vi "vision-board.vi"(8 "error in":errorcluster) -> (0 "error out":errorcluster, 2 "recycle?":bool, 3 "vision board":T2)   [LabVIEW 2019]
uses:
  vision_board_ctl.ctl
panel:
  out "Image Out 3":T1(plugin-control)
  out "Array":string[][](array[string])
  out "Image Out 2":T1(plugin-control)
  out "recycle index":i32
  out "Image Out":T1(plugin-control)
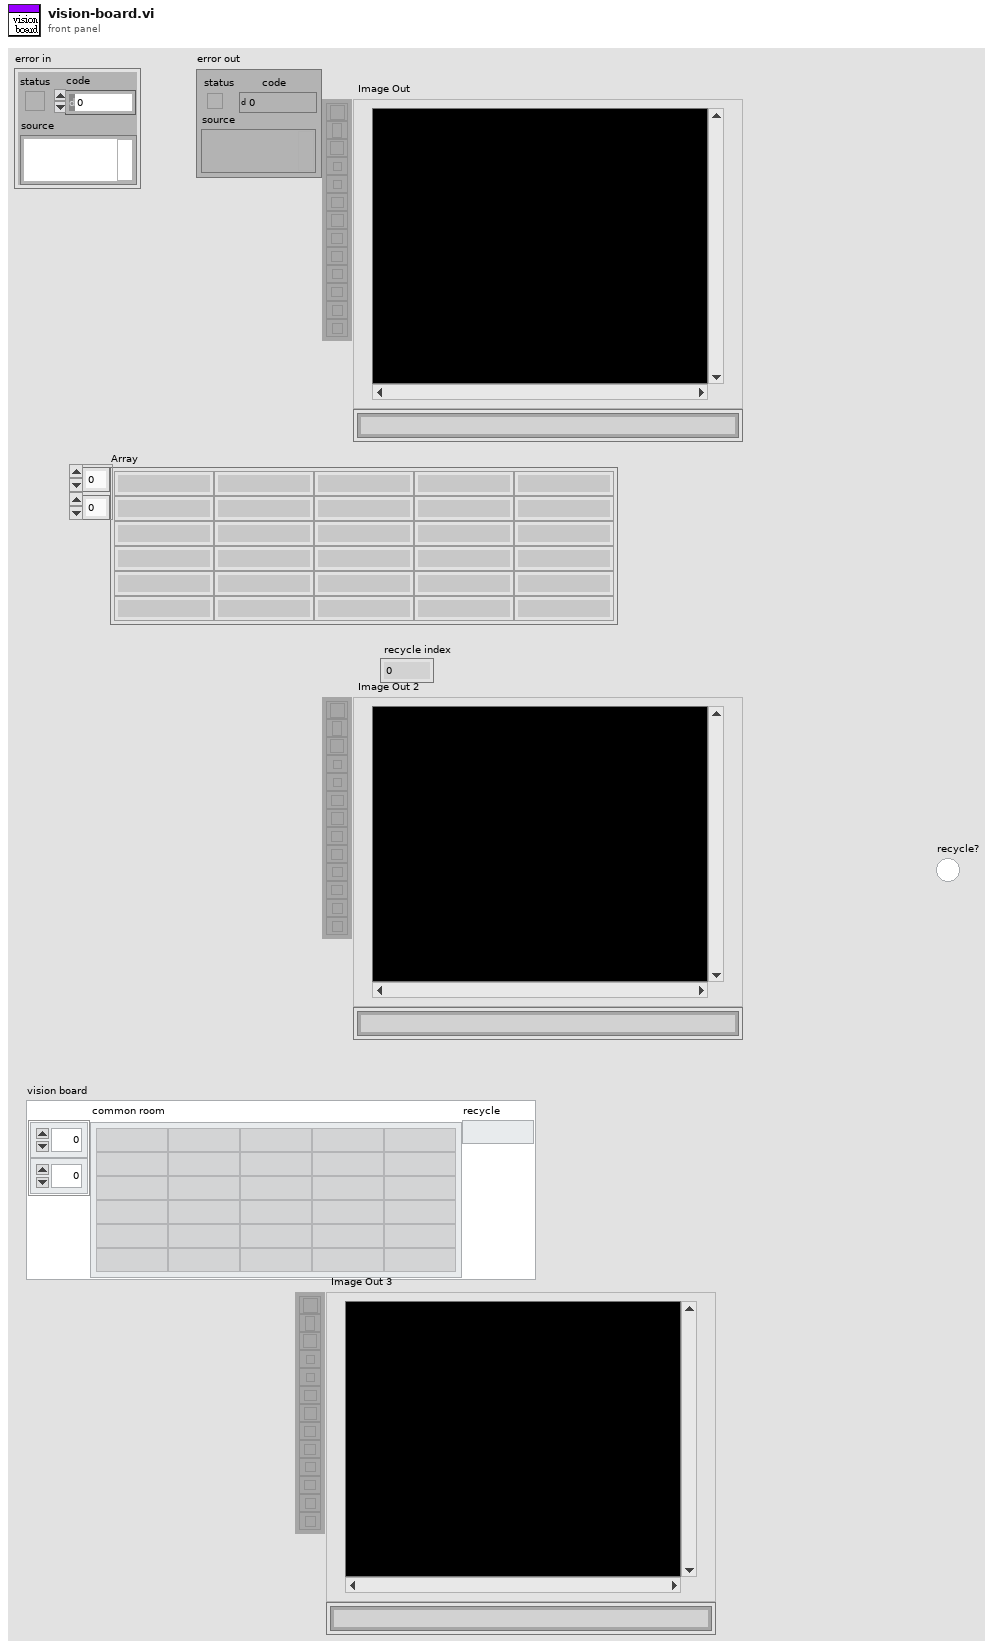
[diagram p1: front panel]
types:
  T1 = typedef "IMAQ Image.ctl" = refnum<image>
  T2 = typedef "vision_board_ctl.ctl" = cluster{"common room":string[][], "recycle":string}
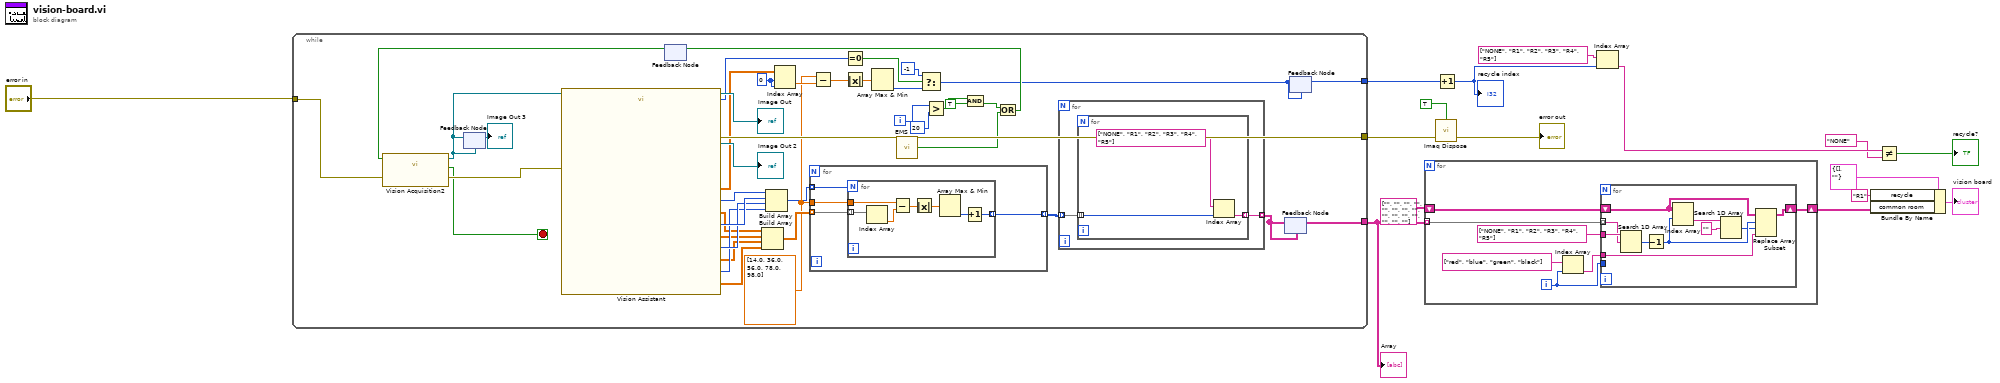
[diagram p0: block diagram]
diagram:
  n1 = while {
    tunnel: [w22] -> w16
    tunnel: "error in" -> [w32]
    tunnel: [w52] -> w4
    tunnel: [w24] -> w15
    i -> [w29]
    stop <- w20 stop-if-true
    w39 = sgl[] [14.0, 36.0, 56.0, 78.0, 98.0] ("Array")
    w55 = 0 ("length")
    n2 = feedback #1() -> (w25:bool)  [unwired: 1 in]
    n3 = call "Vision Acquisition2"("Stop (F)"=w25, "error in"=w32) -> ("Image Out"=w18:T1, "Stopped"=w20:bool, "error out"=w31:errorcluster)  [unwired: 23 in]
    n4 = feedback-in #2(w18) -> ()
    n5 = feedback #2(w18) -> (→"Image Out 3":T1)
    n6 = call "Vision Assistant"("Image In"=w18, "error in"=w31) -> ("Number of Particles (black)"=w45:i32, "Number of Particles (green)"=w46:i32, "Number of Particles (Blue)"=w47:i32, "Number of Particles (red)"=w48:i32, "Image Buffer (Image Buffer 5)"=→"Image Out 2":T1, "Image Out"=→"Image Out":T1, "Number of Particles (Yellow)"=w34:i32, "Particle Measurements (Pixels) (Yellow)"=w38:dbl[][], "Particle Measurements (Pixels) (red)"=w44:dbl[][], "Particle Measurements (Pixels) (Blue)"=w41:dbl[][], "Particle Measurements (Pixels) (green)"=w42:dbl[][], "Particle Measurements (Pixels) (black)"=w43:dbl[][], "error out"=w52:errorcluster)  [unwired: 13 in]
    n7 = Build Array(w44, w41, w42, w43) -> (w40:dbl[][][])
    n8 = Build Array(w48, w47, w46, w45) -> (w33:i32[])
    n9 = Index Array(array=w38, index (row)=w55, index (col)=w55) -> (element=w54:dbl)
    n10 = for {
      tunnel: w33 -> [w66] mode=indexing
      tunnel: w40 -> [w65] mode=indexing
      tunnel: w39 -> [w64]
      tunnel: [w63] -> w35 mode=indexing
      n11 = for {
        N: w66 -> [_]
        tunnel: w65 -> [w73] mode=indexing
        tunnel: w64 -> [w72]
        tunnel: [w67] -> w63 mode=indexing
        n12 = Index Array(array=w73) -> (element=w71:dbl)  [unwired: 1 in]
        n13 = Subtract(x=w72, y=w71) -> (x-y=w69:dbl[])
        n14 = Absolute Value(x=w69) -> (abs(x)=w70:dbl[])
        n15 = Array Max & Min(array=w70) -> (min index (indices)=w68:i32)  [unwired: 3 out]
        n16 = Increment(x=w68) -> (x+1=w67:i32)
      }
    }
    n17 = Subtract(x=w39, y=w54) -> (x-y=w57:dbl[])
    n18 = Equal To 0?(x=w34) -> (x = 0?=w37:bool)
    n19 = Absolute Value(x=w57) -> (abs(x)=w56:dbl[])
    n20 = Array Max & Min(array=w56) -> (min index (indices)=w53:i32)  [unwired: 3 out]
    n21 = call "EMS.vi"() -> ("A/DIO4 (Pin 19)"=w51:bool)
    n22 = Select(t=-1, s=w37, f=w53) -> (s? t:f=w21:i32)
    n23 = Greater?(x=w29, y=20) -> (0:w27:bool)
    n24 = And(x=w27, y=TRUE) -> (x .and. y?=w30:bool)
    n25 = Or(x=w30, y=w51) -> (x .or. y?=w26:bool)
    n26 = feedback-in #1(w26) -> ()
    n27 = for {
      tunnel: w35 -> [w58] mode=indexing
      tunnel: [w59] -> w23 mode=indexing
      n28 = for {
        tunnel: w58 -> [w61] mode=indexing
        tunnel: [w60] -> w59 mode=indexing
        n29 = Index Array(array=string[] ["NONE", "R1", "R2", "R3", "R4", "R5"], index=w61) -> (element=w60:string)
      }
    }
    n30 = feedback-in #3(w23) -> ()
    n31 = feedback #3(w23) -> (w24:string[][])
    n32 = feedback-in #4(w21) -> ()
    n33 = feedback #4(w21) -> (w22:i32)
  }
  "Array" <- w15
  n34 = for {
    tunnel: w15 -> [w80] mode=indexing
    shift-right: [w74] -> w13
    shift-left: string[][] [["", "", ""], ["", "", ""], ["", "", ""], ["", "", ""], ["", "", ""]] -> [w75]
    i -> [w76]
    n35 = Index Array(array=string[] ["red", "blue", "green", "black"], index=w76) -> (element=w77:string)
    n36 = for {
      tunnel: w80 -> [w89] mode=indexing
      tunnel: string[] ["NONE", "R1", "R2", "R3", "R4", "R5"] -> [w90]
      tunnel: w77 -> [w82]
      tunnel: w76 -> [_]
      shift-right: [w81] -> w74
      shift-left: w75 -> [w85]
      n37 = Search 1D Array(1D array=w90, element=w89) -> (index of element=w88:i32)  [unwired: 1 in]
      n38 = Decrement(x=w88) -> (x-1=w84:i32)
      n39 = Index Array(array=w85, index (row)=w84) -> (element=w87:string[])  [unwired: 1 in]
      n40 = Search 1D Array(1D array=w87, element="") -> (index of element=w83:i32)  [unwired: 1 in]
      n41 = Replace Array Subset(array=w85, new element=w82, index (row)=w84, index (col)=w83) -> (w81:string[][])
    }
  }
  n42 = call "Imaq Dispose"("All Images? (No)"=TRUE, "error in (no error)"=w4) -> ("error out"=→"error out":errorcluster)  [unwired: 4 in]
  n43 = Increment(x=w16) -> (x+1=w10:i32)
  "recycle index" <- w10
  n44 = Index Array(array=string[] ["NONE", "R1", "R2", "R3", "R4", "R5"], index=w10) -> (element=w9:string)
  n45 = Bundle By Name(cluster=T2 {"common room"=[], "recycle"=""} ("vision board"), "recycle"="R1", "common room"=w13) -> (→"vision board":T2)
  n46 = Not Equal?(x=w9, y="NONE") -> (x != y?=→"recycle?":bool)
